vi "readFromXML.vi"(8 "error in (no error)":errorcluster, 10 "XML in":string, 11 "TCSWFSCommand in":refnum<class "TCSWFSCommand.lvclass">) -> (0 "error out":errorcluster, 3 "TCSWFSCommand out":refnum<class "TCSWFSCommand.lvclass">)   [LabVIEW 2014, in "TCSDataDefinitions.lvlib" / "TCSWFSCommand.lvlib" / "TCSWFSCommand.lvclass"]
uses:
  TCSWFSCommand.lvclass
  TCSCommand/TCSCommand/TCSCommand.lvclass
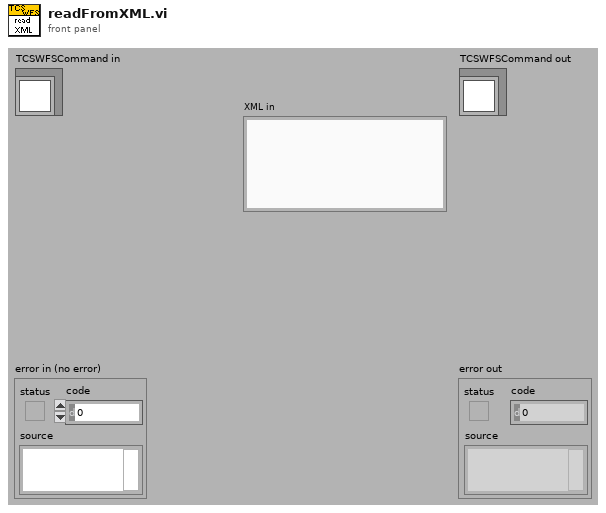
[diagram p1: front panel]
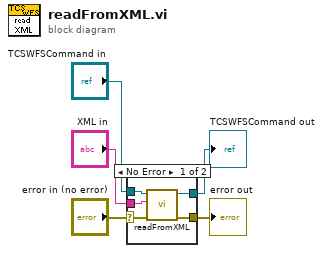
[diagram p0: block diagram]
diagram:
  n1 = case shown="No Error" "error in (no error)" {
    selector: "error in (no error)" -> [w7 w11]
    tunnel: [w6 w11] -> w4
    tunnel: [w9 w12] -> w2
    tunnel: "TCSWFSCommand in" -> [w10 w12]
    tunnel: "XML in" -> [w8 _]
    frame No Error {
      n2 = call-parent "readFromXML.vi"("error in (no error)"=w7, "XML in"=w8, "TCSCommand in"=w10) -> ("error out"=w6:errorcluster, "TCSCommand out"=w9:refnum<class "TCSWFSCommand.lvclass">)  [unwired: 7 in]
    }
    frame Error {
    }
  }
  "error out" <- w4
  "TCSWFSCommand out" <- w2
